vi "Audio Test.Check CL Args.vi"(7 "Simulate":bool, 11 "Sim CL Args":string[](array[string])) -> (1 "Args":string[](array[string]), 2 "Action":string, 3 "CmdLine":bool)   [LabVIEW 2018]
panel:
  out "CL Args":string[](array[string])
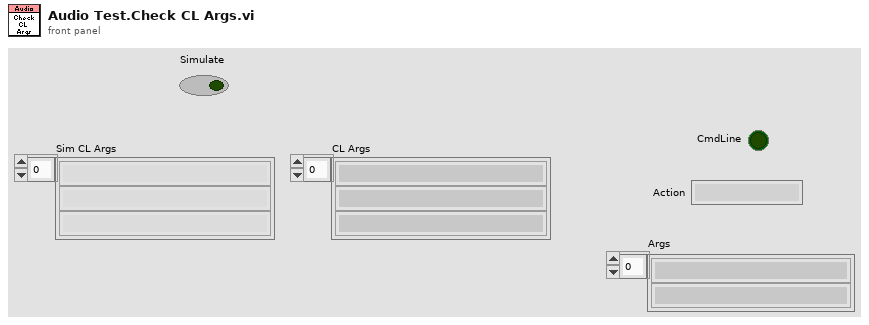
[diagram p1: front panel]
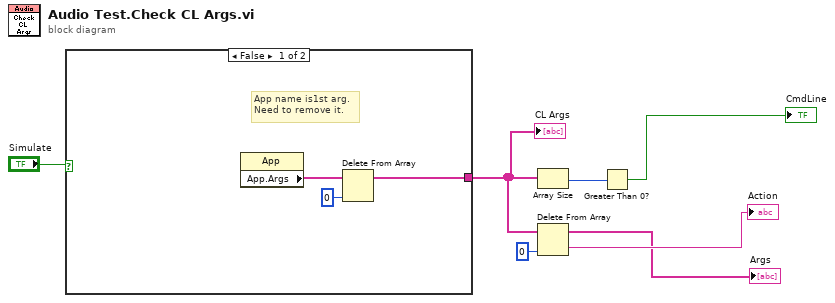
[diagram p0: block diagram]
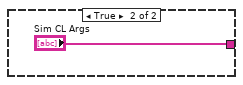
[diagram p2: hidden frame]
diagram:
  n1 = case shown="False" "Simulate" {
    tunnel: [w10 "Sim CL Args"] -> w5
    frame False {
      # "App name is1st arg.\nNeed to remove it."
      n2 = property class="App"() -> ("App.Args"=w8:string[])  [unwired: 2 in, 2 out]
      n3 = Delete From Array(array=w8, index=0) -> (array with subset deleted=w10:string[])  [unwired: 1 in, 1 out]
    }
    frame True {
    }
  }
  "CL Args" <- w5
  n4 = Array Size(array=w5) -> (size(s)=w7:i32)
  n5 = Delete From Array(array=w5, index=0) -> (deleted portion=→"Action":string, array with subset deleted=→"Args":string[])  [unwired: 1 in]
  n6 = Greater Than 0?(x=w7) -> (x > 0?=→"CmdLine":bool)
